vi "CreateObservers.vi"(8 "error in (no error)":errorcluster, 11 "ObserverFactory in":refnum<class "NotificationFactory.lvclass">) -> (0 "error out":errorcluster, 2 "Observers":refnum<class "Notification.lvclass">[](array[class]), 3 "ObserverFactory out":refnum<class "NotificationFactory.lvclass">)   [LabVIEW 2020, in "NotificationFactory.lvclass"]
uses:
  NotificationFactory.lvclass
  Observer/Notification.lvclass
  NotificationFactory.lvclass/NotificationFactory.ctl
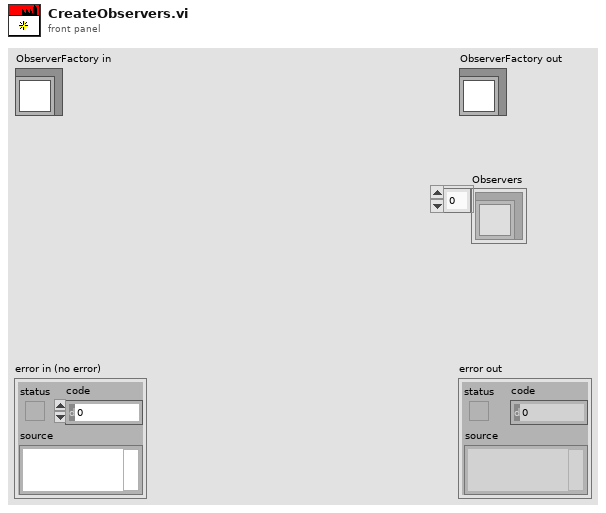
[diagram p1: front panel]
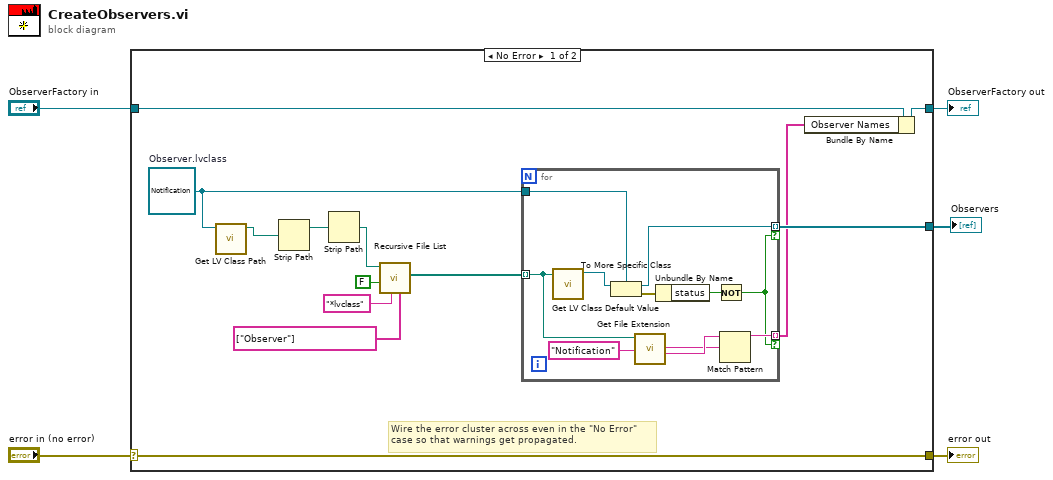
[diagram p0: block diagram]
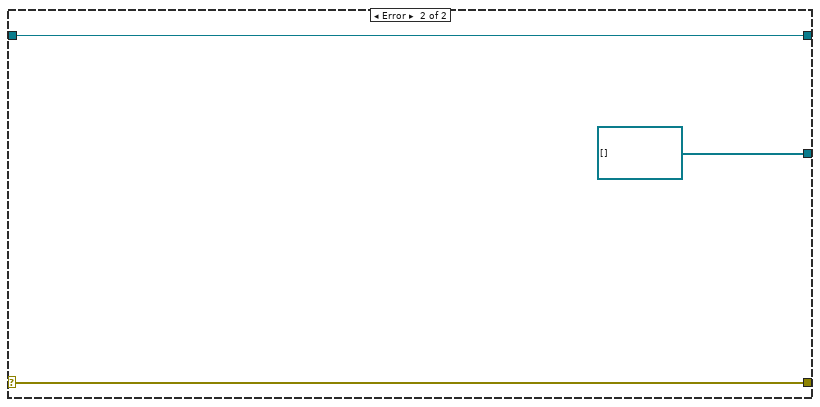
[diagram p2: hidden frame]
diagram:
  n1 = case shown="No Error" "error in (no error)" {
    selector: "error in (no error)" -> [w17 w31]
    tunnel: [w17 w31] -> w4
    tunnel: [w7 w30] -> w2
    tunnel: "ObserverFactory in" -> [w18 w30]
    tunnel: [w8 refnum<class "Notification.lvclass">[] []] -> w1
    frame No Error {
      w12 = refnum<class "Notification.lvclass"> refnum  # Observer.lvclass
      # "Wire the error cluster across even in the \"No Error\"\ncase so that warnings get propagated."
      n2 = call <vilib>:"Get LV Class Path.vi"("object"=w12) -> ("class path"=w14:path)  [unwired: 9 in, 1 out]
      n3 = Strip Path(path=w14) -> (stripped path=w13:path)  [unwired: 1 out]
      n4 = Strip Path(path=w13) -> (stripped path=w16:path)  [unwired: 1 out]
      n5 = call <vilib>:"Recursive File List.vi"("Folders to Exclude"=string[] ["Observer"], "pattern"="*lvclass", "Continue Recursing on Error? (F)"=FALSE, "Folder Path"=w16) -> ("All Files in Dir"=w15:path[])  [unwired: 3 in, 4 out]
      n6 = for {
        tunnel: w15 -> [w21] mode=indexing
        tunnel: w12 -> [w26]
        tunnel: [w25] -> w8 mode=indexing if=w19
        tunnel: [w20] -> w6 mode=indexing if=w19
        n7 = call <vilib>:"Get LV Class Default Value.vi"("class path"=w21) -> ("object"=w28:refnum<class>)  [unwired: 9 in, 1 out]
        n8 = To More Specific Class(target class=w26, reference=w28) -> (specific class reference=w25:refnum<class "Notification.lvclass">, error out=w24:errorcluster)  [unwired: 1 in]
        n9 = call <vilib>:"Get File Extension.vi"("file"=w21) -> ("filename without extension"=w23:string)  [unwired: 6 in, 4 out]
        n10 = Unbundle By Name(w24) -> ("status"=w27:bool)
        n11 = Not(x=w27) -> (.not. x?=w19:bool)
        n12 = Match Pattern(string=w23, regular expression="Notification") -> (before substring=w20:string)  [unwired: 1 in, 3 out]
      }
      n13 = Bundle By Name(cluster=w18, "Observer Names"=w6) -> (w7:refnum<class "NotificationFactory.lvclass">)
    }
    frame Error {
    }
  }
  "error out" <- w4
  "ObserverFactory out" <- w2
  "Observers" <- w1
